vi "发送读取接收事件引用.vi"(7 "Message Priority (Normal)":T1=enum."Normal" caption="消息优先级（标准）", 8 "error in (no error)":errorcluster caption="错误输入（无错误）", 10 "timeout in ms (-1)":i32=-1 caption="超时毫秒(-1)", 11 "Message Enqueuer":refnum<class "Message Enqueuer.lvclass"> caption="消息待入队列") -> (0 "error out":errorcluster caption="错误输出", 1 "timed out?":bool caption="超时？", 2 "接收事件引用":refnum<user-event>, 3 "Message Enqueuer out":refnum<class "Message Enqueuer.lvclass"> caption="消息待入队列输出")   [LabVIEW 2015, in "上位机.lvlib" / "读取接收事件引用消息.lvclass"]
doc: "本VI将消息发送至操作者。"
uses:
  <vilib>/ActorFramework/Reply Msg/Reply Msg.lvclass
  <vilib>/ActorFramework/Message Enqueuer/Message Enqueuer.lvclass
  <vilib>/ActorFramework/Message Enqueuer/Message Priority.ctl
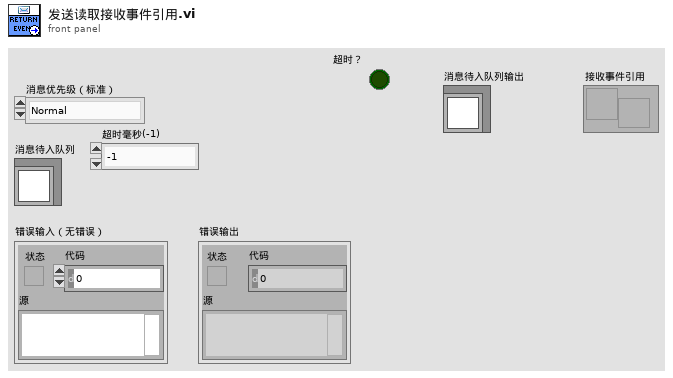
[diagram p1: front panel]
types:
  T1 = typedef "Actor Framework.lvlib/Message Enqueuer.lvclass/Message Priority.ctl" = enum16{"Low", "Normal", "High"}
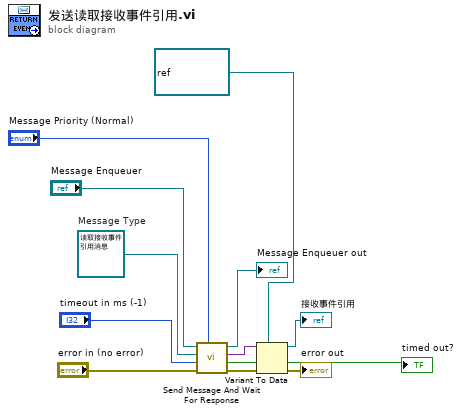
[diagram p0: block diagram]
diagram:
  w11 = refnum<class "读取接收事件引用消息.lvclass"> refnum  # Message Type
  n1 = call <vilib>:"Send Message And Wait For Response.vi"("Message Priority (Normal)"="Message Priority (Normal)", "error in (no error)"="error in (no error)", "timeout in ms (-1)"="timeout in ms (-1)", "Original Message"=w11, "Message Enqueuer in"="Message Enqueuer") -> ("error out"=w3:errorcluster, "timed out?"=→"timed out?":bool, "Reply"=w6:variant, "Message Enqueuer out"=→"Message Enqueuer out":refnum<class "Message Enqueuer.lvclass">)  [unwired: 3 in]
  n2 = Variant To Data(error in=w3, type=refnum<user-event> refnum ("发送数据用户事件"), Variant=w6) -> (data=→"接收事件引用":refnum<user-event>, error out=→"error out":errorcluster)
